vi "FPGA是否采集全局.vi"() -> ()   [LabVIEW 2013]
panel:
  out "是否采集数据":bool
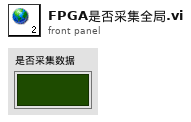
[diagram p1: front panel]
diagram:
